vi "Initialize Logger.vi"(11 "error in":errorcluster) -> (4 "event data":T1, 15 "error out":errorcluster)   [LabVIEW 2021, in "Event Logger.lvlib"]
uses:
  Event Logger.lvlib
  TypeDefs/Event Data Cluster.ctl
  TypeDefs/Event Values.ctl
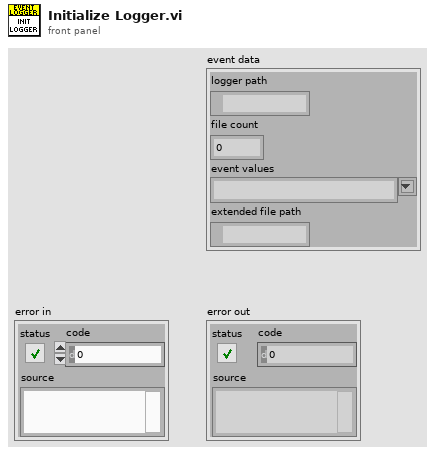
[diagram p1: front panel]
types:
  T1 = typedef "Event Logger.lvlib/Event Data Cluster.ctl" = cluster{"logger path":path, "file count":i32, "event values":T2, "extended file path":path}
  T2 = typedef "Event Logger.lvlib/Event Values.ctl" = string
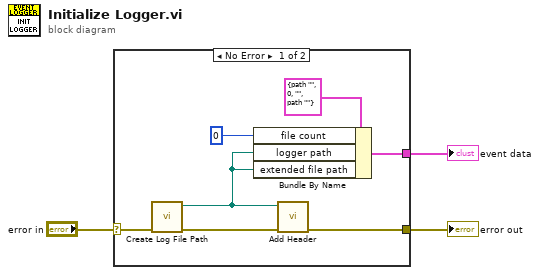
[diagram p0: block diagram]
diagram:
  n1 = case shown="No Error" "error in" {
    selector: "error in" -> [w10 w11]
    tunnel: [w9 w11] -> w2
    tunnel: [w5 _] -> w1
    frame No Error {
      n2 = call "Create Log File Path.vi"("error in"=w10) -> ("error out"=w7:errorcluster, "logger path"=w4:path)  [unwired: 9 in]
      n3 = Bundle By Name(cluster=T1 {"logger path"=path "", "file count"=0, "event values"="", "extended file path"=path ""} ("EventData"), "file count"=0 ("FileCount"), "logger path"=w4, "extended file path"=w4) -> (w5:T1)
      n4 = call "Add Header.vi"("error in"=w7, "logger path"=w4) -> ("error out"=w9:errorcluster)  [unwired: 9 in]
    }
    frame Error {
    }
  }
  "error out" <- w2
  "event data" <- w1
